vi "APS get gantry param.vi"(7 "ParaDat":i32, 8 "error in (no error)":errorcluster caption="错误输入（无错误）", 9 "ParaNum":i32, 10 "GroupNum":i32, 11 "Board_ID":i32) -> (0 "error out":errorcluster caption="错误输出", 3 "function return":i32, 5 "ParaDat out":i32)   [LabVIEW 2011, in "APS168.lvlib"]
doc: "I32 FNTYPE APS_get_gantry_param( I32 Board_ID, I32 GroupNum, I32 ParaNum, I32 *ParaDat );"
uses:
  APS168.lvlib
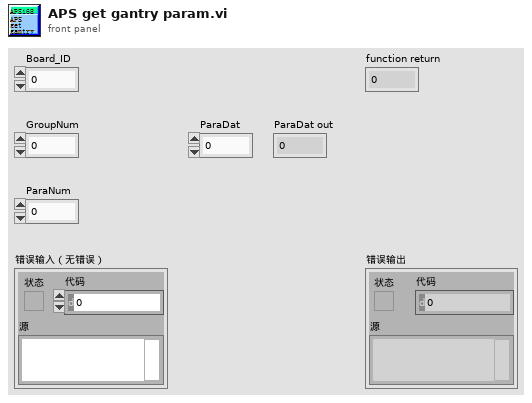
[diagram p1: front panel]
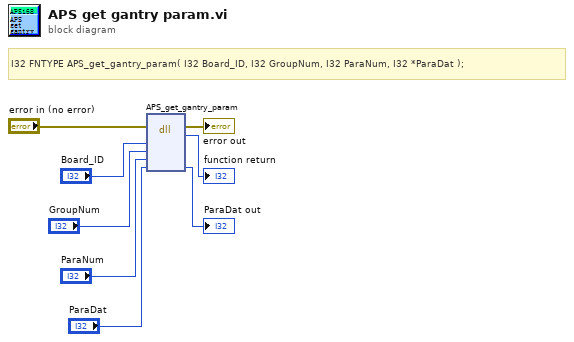
[diagram p0: block diagram]
diagram:
  # "I32 FNTYPE APS_get_gantry_param( I32 Board_ID, I32 GroupNum, I32 ParaNum, I32 *ParaDat );"
  n1 = dll-call lib="PTH1Labs E软件ADLINK 204CAPS_1_7_1_LIB line 连续运动204APS168.*" fn="APS_get_gantry_param"(error in="error in (no error)", "Board_ID"="Board_ID", "GroupNum"="GroupNum", "ParaNum"="ParaNum", "ParaDat"="ParaDat") -> (error out=→"error out":errorcluster, →"function return":i32, "ParaDat"=→"ParaDat out":i32)  [unwired: 5 in, 1 out]
